vi "FTW-ERR-Ignore.vi"(9 "Error Code":i32, 11 "error in":errorcluster) -> (15 "error out":errorcluster)   [LabVIEW 2015]
doc: "Throws an error if the \"Error Code\" input is non-zero."
panel:
  # "Inputs"
  # "Outputs"
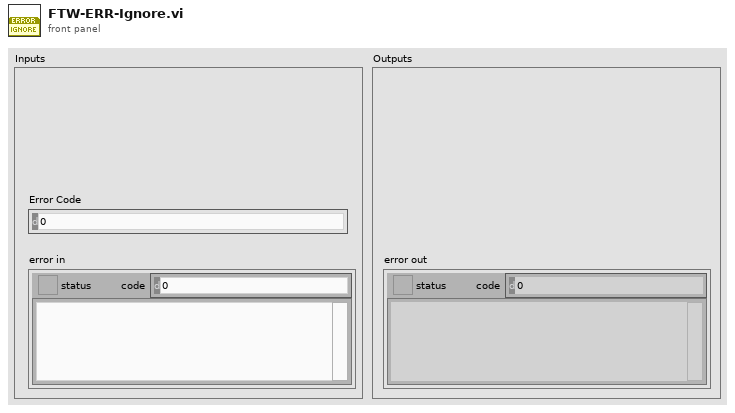
[diagram p1: front panel]
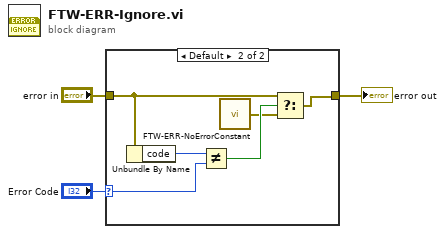
[diagram p0: block diagram]
diagram:
  n1 = case shown="Default" "Error Code" {
    selector: "Error Code" -> [_ w9]
    tunnel: "error in" -> [w4 w6]
    tunnel: [w4 w5] -> w2
    frame 0 {
    }
    frame Default {
      n2 = Unbundle By Name(w6) -> ("code"=w10:i32)
      n3 = Not Equal?(x=w10, y=w9) -> (x != y?=w8:bool)
      n4 = call "FTW-ERR-NoErrorConstant.vi"() -> ("no error"=w7:errorcluster)
      n5 = Select(t=w6, s=w8, f=w7) -> (s? t:f=w5:errorcluster)
    }
  }
  "error out" <- w2
